vi "createInitArray.vi"(9 "timeAxisLim":dbl, 10 "sampling rate [kHz]":dbl, 11 "Channels to read":i32) -> (2 "Numeric":i32, 3 "Array":dbl[][](array[numeric]))   [LabVIEW 2024]
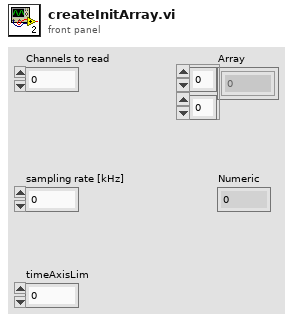
[diagram p1: front panel]
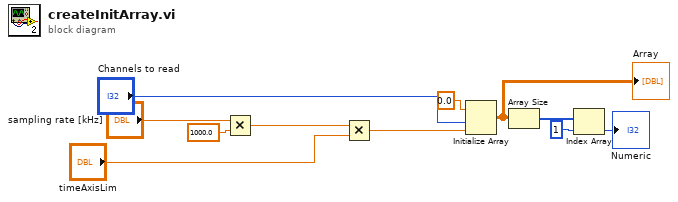
[diagram p0: block diagram]
diagram:
  n1 = Multiply(x="sampling rate [kHz]", y=1000.0) -> (x*y=w4:dbl)
  n2 = Multiply(x=w4, y="timeAxisLim") -> (x*y=w6:dbl)
  n3 = Initialize Array(0.0 ("element"), "Channels to read", w6) -> (w2:dbl[][])
  "Array" <- w2
  n4 = Array Size(array=w2) -> (size(s)=w1:i32[])
  n5 = Index Array(array=w1, index=1) -> (element=→"Numeric":i32)
